vi "acq.Average.vi"(4 "jpg?":bool, 5 "flip":T1, 6 "Save":bool, 7 "path":T2, 8 "error in":errorcluster, 9 "Dark":u16[][](array[numeric]), 10 "PL":u16[][](array[numeric]), 11 "Bright":u16[][](array[numeric])) -> (0 "error out":errorcluster, 2 "PL":u16[][](array[numeric]), 3 "IL":u16[][](array[numeric]))   [LabVIEW 2020]
uses:
  _controls/path.ctl
  _controls/flip.ctl
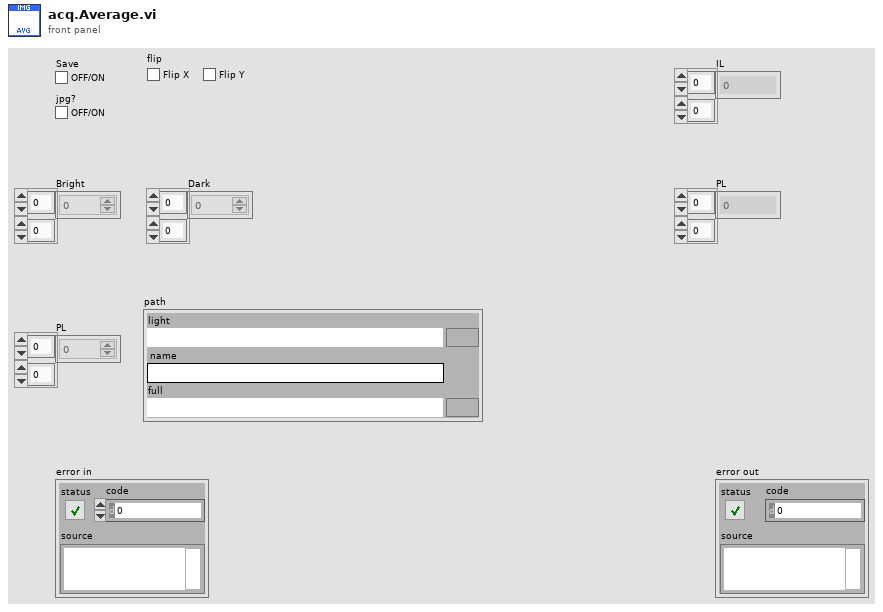
[diagram p1: front panel]
types:
  T1 = typedef "flip.ctl" = cluster{"x":bool, "y":bool}
  T2 = typedef "path.ctl" = cluster{"light":path, "name":string, "full":path}
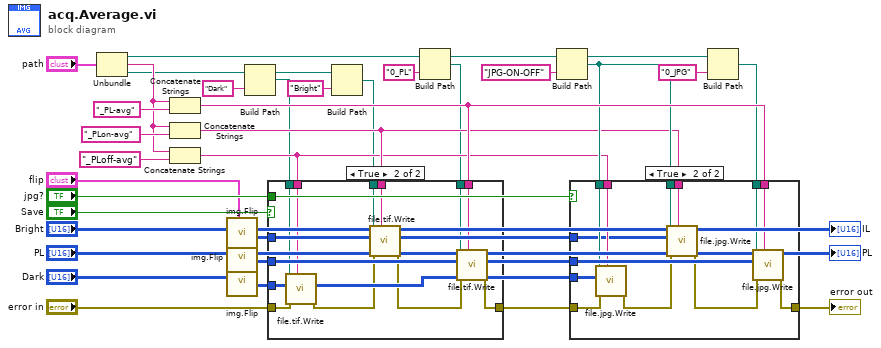
[diagram p0: block diagram]
diagram:
  n1 = Unbundle("path") -> ("light"=w10:path, "name"=w16:string, "full"=w14:path)
  n2 = Concatenate Strings(w16, "_PL-avg" ("name or relative path")) -> (w26:string)
  n3 = Concatenate Strings(w16, "_PLon-avg" ("name or relative path")) -> (w21:string)
  n4 = Concatenate Strings(w16, "_PLoff-avg" ("name or relative path")) -> (w20:string)
  n5 = call "img.Flip.vi"("flip"="flip", "image in"="Bright") -> ("image out"=w6:u16[][])  [unwired: 9 in]
  n6 = call "img.Flip.vi"("flip"="flip", "image in"="PL") -> ("image out"=w8:u16[][])  [unwired: 9 in]
  n7 = call "img.Flip.vi"("flip"="flip", "image in"="Dark") -> ("image out"=w7:u16[][])  [unwired: 9 in]
  n8 = Build Path(base path=w14, name or relative path="Dark") -> (appended path=w12:path)
  n9 = Build Path(base path=w14, name or relative path="Bright") -> (appended path=w13:path)
  n10 = Build Path(base path=w10, name or relative path="0_PL") -> (appended path=w9:path)
  n11 = case shown="True" "Save" {
    tunnel: w6 -> [_ w46]
    tunnel: [w33 w45] -> w28
    tunnel: w8 -> [_ w44]
    tunnel: w7 -> [_ w41]
    tunnel: w12 -> [_ w40]
    tunnel: w13 -> [_ w39]
    tunnel: "error in" -> [w33 w38]
    tunnel: "jpg?" -> [_ _]
    tunnel: w26 -> [_ w37]
    tunnel: w21 -> [_ w36]
    tunnel: w20 -> [_ w35]
    tunnel: w9 -> [_ w34]
    frame False {
    }
    frame True {
      n12 = call "file.tif.Write.vi"("name"=w35, "error in"=w38, "u16 pixmap"=w41, "path"=w40) -> ("error out"=w43:errorcluster)  [unwired: 7 in]
      n13 = call "file.tif.Write.vi"("name"=w36, "error in"=w43, "u16 pixmap"=w46, "path"=w39) -> ("error out"=w42:errorcluster)  [unwired: 7 in]
      n14 = call "file.tif.Write.vi"("name"=w37, "error in"=w42, "u16 pixmap"=w44, "path"=w34) -> ("error out"=w45:errorcluster)  [unwired: 7 in]
    }
  }
  n15 = Build Path(base path=w10, name or relative path="JPG-ON-OFF") -> (appended path=w22:path)
  n16 = Build Path(base path=w10, name or relative path="0_JPG") -> (appended path=w18:path)
  n17 = case shown="True" "jpg?" {
    tunnel: [w47 w60] -> w27
    tunnel: w8 -> [_ w59]
    tunnel: w18 -> [_ w58]
    tunnel: w7 -> [_ w55]
    tunnel: w22 -> [_ w54]
    tunnel: w22 -> [_ w53]
    tunnel: w28 -> [w47 w52]
    tunnel: w26 -> [_ w51]
    tunnel: w21 -> [_ w50]
    tunnel: w20 -> [_ w49]
    tunnel: w6 -> [_ w48]
    frame False {
    }
    frame True {
      n18 = call "file.jpg.Write.vi"("name"=w49, "error in"=w52, "u16 pixmap"=w55, "path"=w54) -> ("error out"=w57:errorcluster)  [unwired: 7 in]
      n19 = call "file.jpg.Write.vi"("name"=w50, "error in"=w57, "u16 pixmap"=w48, "path"=w53) -> ("error out"=w56:errorcluster)  [unwired: 7 in]
      n20 = call "file.jpg.Write.vi"("name"=w51, "error in"=w56, "u16 pixmap"=w59, "path"=w58) -> ("error out"=w60:errorcluster)  [unwired: 7 in]
    }
  }
  "error out" <- w27
  "PL" <- "PL"
  "IL" <- "Bright"
